vi "Fetch Multiple.vi"(8 "error in (no error)":errorcluster, 11 "SMU in":refnum<class "NI SMU.lvclass">) -> (0 "error out":errorcluster, 2 "Data":variant, 3 "SMU out":refnum<class "NI SMU.lvclass">)   [LabVIEW 2020, in "NI SMU.lvlib" / "NI SMU.lvclass"]
uses:
  NI SMU.lvclass
  NI SMU.lvclass/NI SMU.ctl
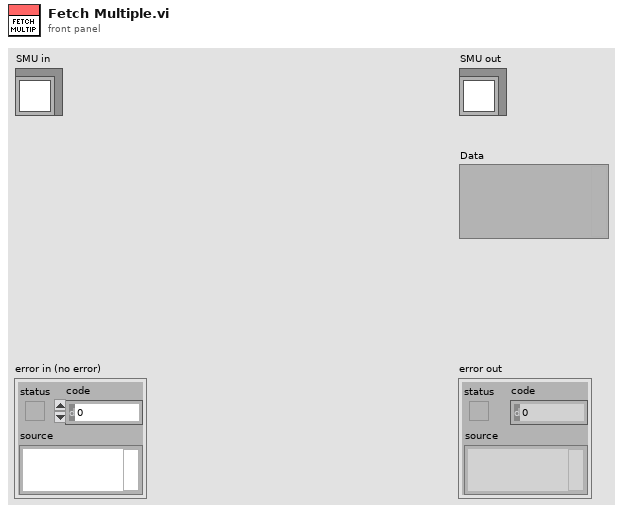
[diagram p1: front panel]
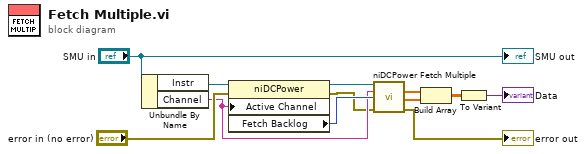
[diagram p0: block diagram]
diagram:
  n1 = Unbundle By Name("SMU in") -> ("Instr"=w11:refnum<k15>, "Channel"=w6:string)
  n2 = property class="niDCPower"(reference=w11, error in="error in (no error)", "Active Channel"=w6) -> (reference out=w9:refnum<k15>, error out=w5:errorcluster, "Fetch Backlog"=w8:i32)
  n3 = call <instrlib>:"niDCPower Fetch Multiple.vi"("instrument handle"=w9, "channel name"=w6, "count (1)"=w8, "error in (no error)"=w5) -> ("voltage measurements"=w4:dbl[], "current measurements"=w3:dbl[], "error out"=→"error out":errorcluster)  [unwired: 6 in, 3 out]
  n4 = Build Array(w4, w3) -> (w2:dbl[][])
  n5 = To Variant(anything=w2) -> (Variant=→"Data":variant)
  "SMU out" <- "SMU in"
